vi "assert null.vi"(8 "error in (no error)":errorcluster, 11 "JSON Value in":refnum<class "JSON Value.lvclass">) -> (0 "error out":errorcluster, 3 "JSON Value out":refnum<class "JSON Value.lvclass">)   [LabVIEW 2016, in "JSON Value.lvclass"]
uses:
  JSON Value.lvclass
  JSON Types.ctl
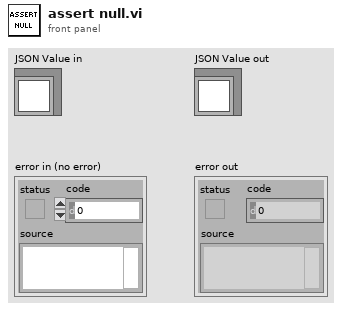
[diagram p1: front panel]
types:
  T1 = typedef "JSON Value.lvclass/JSON Types.ctl" = enum8{"String", "Numeric", "Boolean", "NULL", "Object", "Array"}
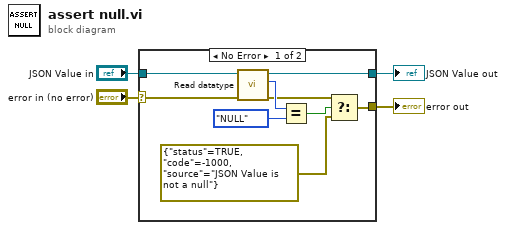
[diagram p0: block diagram]
diagram:
  n1 = case shown="No Error" "error in (no error)" {
    selector: "error in (no error)" -> [w12 w15]
    tunnel: [w6 w15] -> w3
    tunnel: [w11 w14] -> w1
    tunnel: "JSON Value in" -> [w13 w14]
    frame No Error {
      n2 = call "Read datatype.vi"("error in (no error)"=w12, "JSON Value in"=w13) -> ("error out"=w7:errorcluster, "datatype"=w10:T1, "JSON Value out"=w11:refnum<class "JSON Value.lvclass">)  [unwired: 7 in]
      n3 = Equal?(x=w10, y=JSON_Types."NULL") -> (x = y?=w8:bool)
      n4 = Select(t=w7, s=w8, f=errorcluster {"status"=TRUE, "code"=-1000, "source"="JSON Value is not a null"}) -> (s? t:f=w6:errorcluster)
    }
    frame Error {
    }
  }
  "error out" <- w3
  "JSON Value out" <- w1
